vi "Day04-04_텍스트 파일 및 폴더 경로 설정.vi"() -> ()   [LabVIEW 2021]
uses:
  <vilib>/Utility/sysdir.llb/System Directory Type.ctl
panel:
  out "배열":dbl[][](array[numeric])
  out "텍스트 파일 열기 경로":path
  out "텍스트 파일 쓰기 경로":path
  out "파일 경로":path
  out "추가된 경로":path
  out "system directory":path caption="시스템 디렉토리"
  out "Application Directory":path caption="어플리케이션 디렉토리"
  out "경로":path
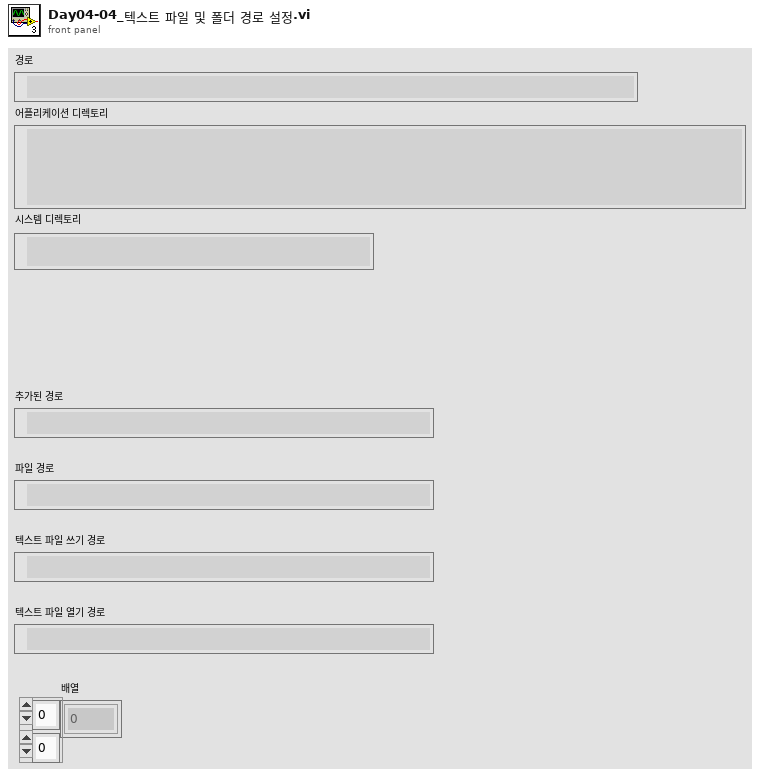
[diagram p1: front panel]
types:
  T1 = enum16{"open", "replace", "create", "open or create", "replace or create", "replace or create with confirmation"}
  T2 = typedef "System Directory Type.ctl" = i32
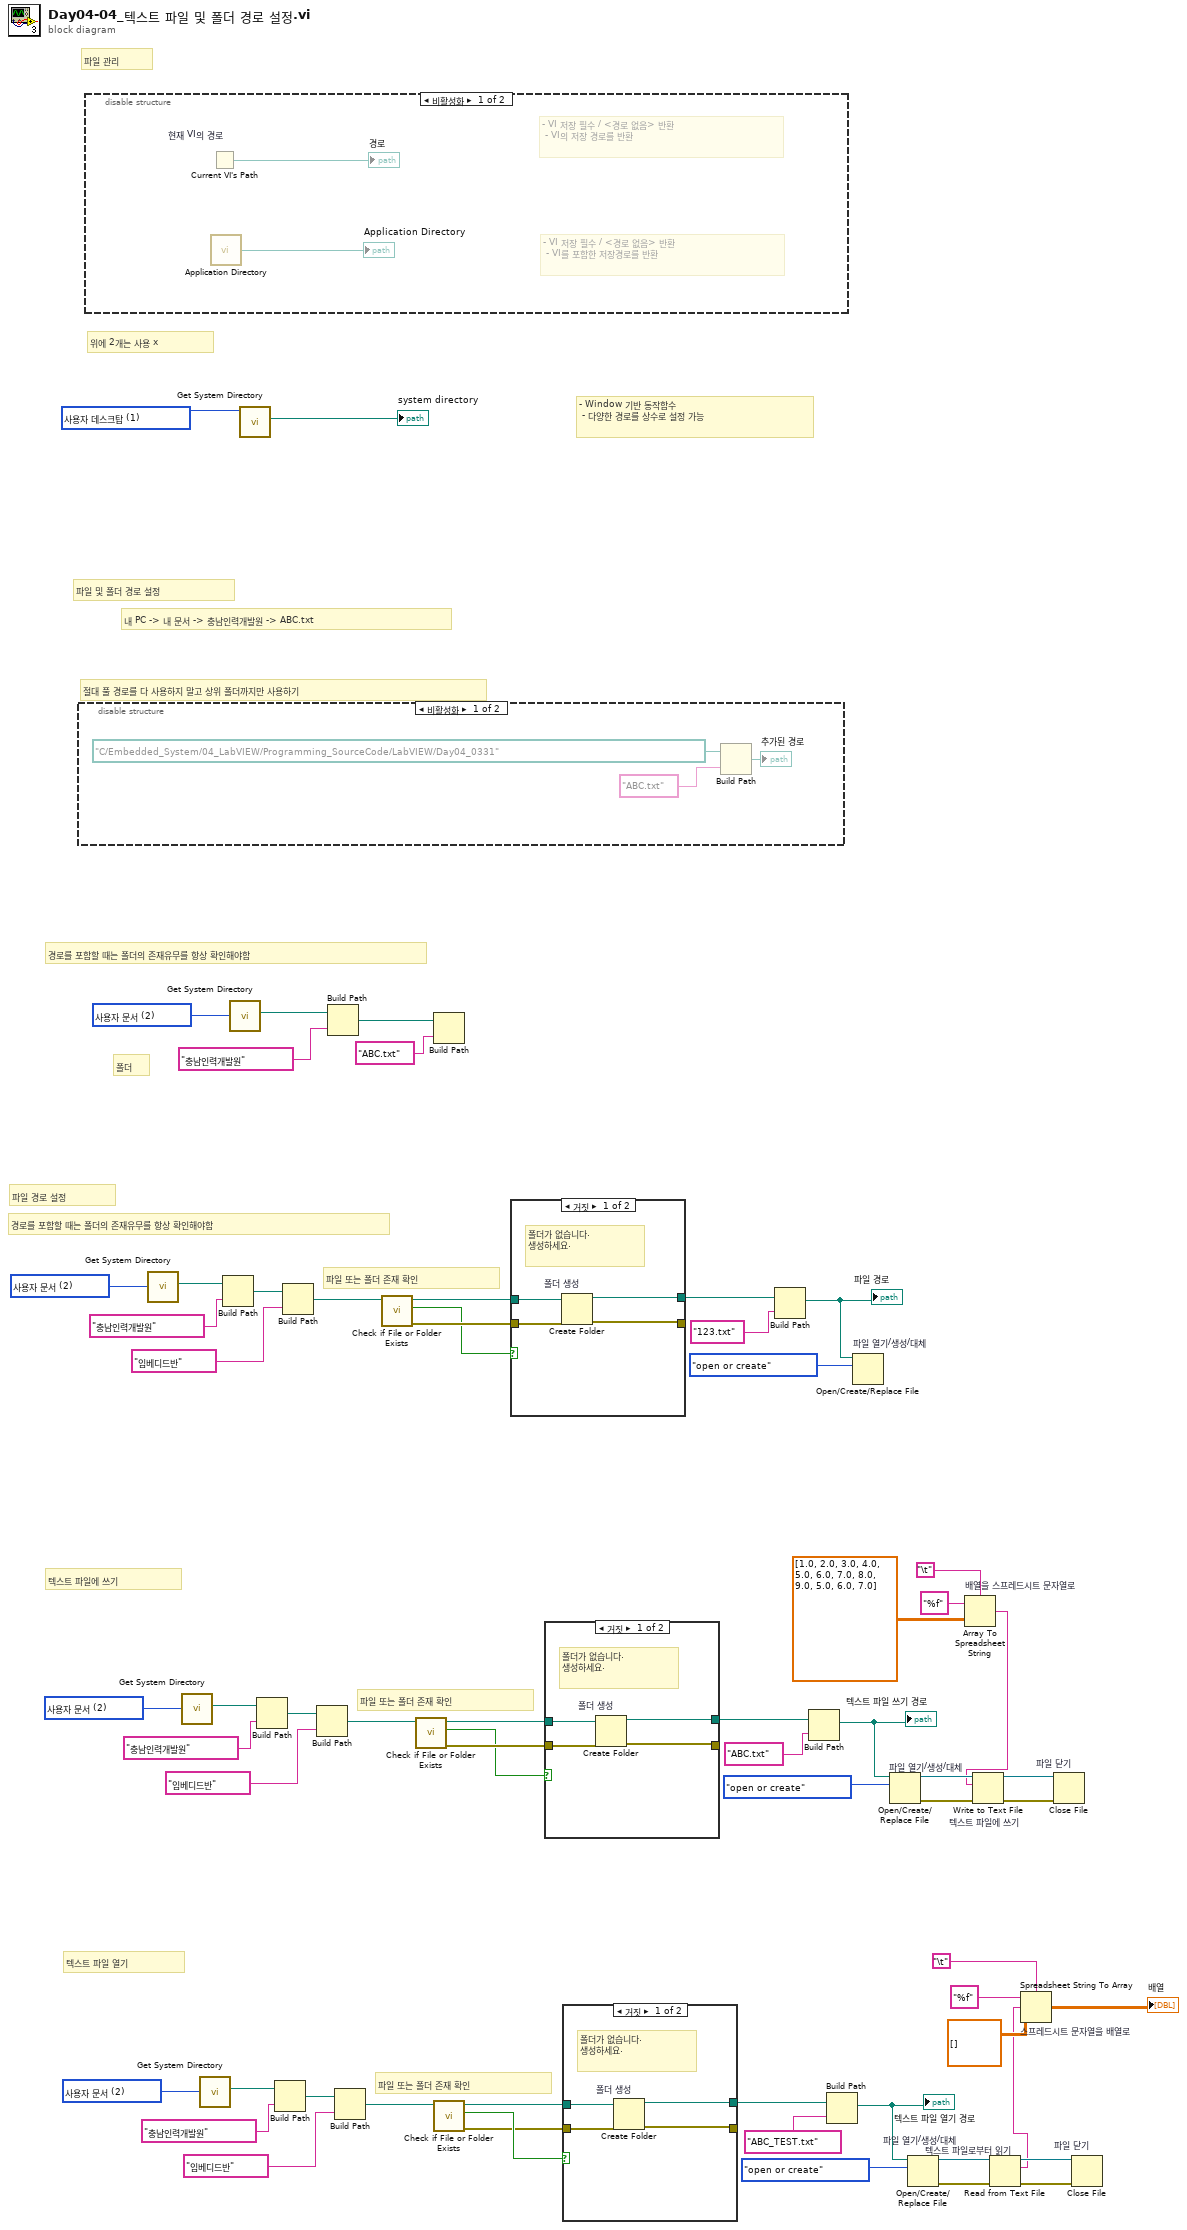
[diagram p0: block diagram]
diagram:
  w10 = T2 2 items=["사용자 홈"=0, "사용자 데스크탑"=1, "사용자 문서"=2, "사용자 어플리케이션 데이터"=3, "사용자 환경"=4, "사용자 임시"=5, "퍼블릭 문서"=6, "퍼블릭 어플리케이션 데이터"=7, "퍼블릭 환경"=8, "퍼블릭 캐시"=13, "시스템 코어 라이브러리"=9, "시스템 설치된 라이브러리"=10, "어플리케이션 파일"=11, "부팅 볼륨 루트"=12] ("system directory type")
  w43 = T2 2 items=["사용자 홈"=0, "사용자 데스크탑"=1, "사용자 문서"=2, "사용자 어플리케이션 데이터"=3, "사용자 환경"=4, "사용자 임시"=5, "퍼블릭 문서"=6, "퍼블릭 어플리케이션 데이터"=7, "퍼블릭 환경"=8, "퍼블릭 캐시"=13, "시스템 코어 라이브러리"=9, "시스템 설치된 라이브러리"=10, "어플리케이션 파일"=11, "부팅 볼륨 루트"=12] ("system directory type")
  w56 = T2 2 items=["사용자 홈"=0, "사용자 데스크탑"=1, "사용자 문서"=2, "사용자 어플리케이션 데이터"=3, "사용자 환경"=4, "사용자 임시"=5, "퍼블릭 문서"=6, "퍼블릭 어플리케이션 데이터"=7, "퍼블릭 환경"=8, "퍼블릭 캐시"=13, "시스템 코어 라이브러리"=9, "시스템 설치된 라이브러리"=10, "어플리케이션 파일"=11, "부팅 볼륨 루트"=12] ("system directory type")
  w61 = T2 2 items=["사용자 홈"=0, "사용자 데스크탑"=1, "사용자 문서"=2, "사용자 어플리케이션 데이터"=3, "사용자 환경"=4, "사용자 임시"=5, "퍼블릭 문서"=6, "퍼블릭 어플리케이션 데이터"=7, "퍼블릭 환경"=8, "퍼블릭 캐시"=13, "시스템 코어 라이브러리"=9, "시스템 설치된 라이브러리"=10, "어플리케이션 파일"=11, "부팅 볼륨 루트"=12] ("system directory type")
  w62 = T2 1 items=["사용자 홈"=0, "사용자 데스크탑"=1, "사용자 문서"=2, "사용자 어플리케이션 데이터"=3, "사용자 환경"=4, "사용자 임시"=5, "퍼블릭 문서"=6, "퍼블릭 어플리케이션 데이터"=7, "퍼블릭 환경"=8, "퍼블릭 캐시"=13, "시스템 코어 라이브러리"=9, "시스템 설치된 라이브러리"=10, "어플리케이션 파일"=11, "부팅 볼륨 루트"=12] ("system directory type")
  # "파일 또는 폴더 존재 확인"
  # "텍스트 파일 열기"
  # "파일 또는 폴더 존재 확인"
  # "텍스트 파일에 쓰기"
  # "파일 경로 설정"
  # "경로를 포함할 때는 폴더의 존재유무를 항상 확인해야함"
  # "파일 또는 폴더 존재 확인"
  # "폴더"
  # "경로를 포함할 때는 폴더의 존재유무를 항상 확인해야함"
  # "절대 풀 경로를 다 사용하지 말고 상위 폴더까지만 사용하기"
  # "내 PC -> 내 문서 -> 충남인력개발원 -> ABC.txt"
  # "파일 및 폴더 경로 설정"
  # "위에 2개는 사용 x"
  # "- Window 기반 동작함수\n - 다양한 경로를 상수로 설정 가능"
  # "파일 관리"
  n1 = disable-structure shown="비활성화" {
    frame Disabled {
      n2 = Build Path(base path=path "C:/Embedded_System/04_LabVIEW/Programming_SourceCode/LabVIEW/Day04_0331" ("이름 또는 상대 경로"), name or relative path="ABC.txt") -> (appended path=→"추가된 경로":path)
    }
    frame Enabled {
    }
  }
  n3 = disable-structure shown="비활성화" {
    frame Disabled {
      # "- VI 저장 필수 / <경로 없음> 반환\n - VI를 포함한 저장경로를 반환"
      # "- VI 저장 필수 / <경로 없음> 반환\n - VI의 저장 경로를 반환"
      n4 = Current VI's Path "현재 VI의 경로"() -> (path=→"경로":path)
      n5 = call <vilib>:"Application Directory.vi"() -> ("Application Directory"=→"Application Directory":path)
    }
    frame Enabled {
    }
  }
  n6 = call <vilib>:"Get System Directory.vi"("system directory type"=w56) -> ("system directory"=w55:path)  [unwired: 10 in]
  n7 = call <vilib>:"Get System Directory.vi"("system directory type"=w43) -> ("system directory"=w42:path)  [unwired: 10 in]
  n8 = call <vilib>:"Get System Directory.vi"("system directory type"=w10) -> ("system directory"=w11:path)  [unwired: 10 in]
  n9 = Build Path(base path=w55, name or relative path="충남인력개발원") -> (appended path=w46:path)
  n10 = call <vilib>:"Get System Directory.vi"("system directory type"=w61) -> ("system directory"=w60:path)  [unwired: 10 in]
  n11 = call <vilib>:"Get System Directory.vi"("system directory type"=w62) -> ("system directory"=→"system directory":path)  [unwired: 10 in]
  n12 = Build Path(base path=w42, name or relative path="충남인력개발원") -> (appended path=w33:path)
  n13 = Build Path(base path=w11, name or relative path="충남인력개발원") -> (appended path=w20:path)
  n14 = Build Path(base path=w46, name or relative path="임베디드반") -> (appended path=w44:path)
  n15 = Build Path(base path=w33, name or relative path="임베디드반") -> (appended path=w31:path)
  n16 = Build Path(base path=w60, name or relative path="충남인력개발원") -> (appended path=w58:path)
  n17 = Build Path(base path=w20, name or relative path="임베디드반") -> (appended path=w22:path)
  n18 = call <vilib>:"Check if File or Folder Exists.vi"("path"=w44) -> ("error out"=w52:errorcluster, "file or folder exists?"=w47:bool, "dup path"=w53:path)  [unwired: 8 in]
  n19 = call <vilib>:"Check if File or Folder Exists.vi"("path"=w31) -> ("error out"=w39:errorcluster, "file or folder exists?"=w34:bool, "dup path"=w40:path)  [unwired: 8 in]
  n20 = Build Path(base path=w58, name or relative path="ABC.txt") -> ()  [unwired: 1 out]
  n21 = call <vilib>:"Check if File or Folder Exists.vi"("path"=w22) -> ("error out"=w14:errorcluster, "file or folder exists?"=w19:bool, "dup path"=w13:path)  [unwired: 8 in]
  n22 = case shown="거짓" w47 {
    tunnel: w53 -> [w72 w74]
    tunnel: w52 -> [w71 w73]
    tunnel: [w70 w74] -> w50
    tunnel: [w69 w73] -> _
    frame False {
      # "폴더가 없습니다.\n생성하세요."
      n23 = Create Folder "폴더 생성"(path (use dialog)=w72, error in=w71) -> (created path=w70:path, error out=w69:errorcluster)  [unwired: 1 in, 1 out]
    }
    frame True {
    }
  }
  n24 = case shown="거짓" w34 {
    tunnel: w40 -> [w78 w80]
    tunnel: w39 -> [w77 w79]
    tunnel: [w76 w80] -> w37
    tunnel: [w75 w79] -> _
    frame False {
      # "폴더가 없습니다.\n생성하세요."
      n25 = Create Folder "폴더 생성"(path (use dialog)=w78, error in=w77) -> (created path=w76:path, error out=w75:errorcluster)  [unwired: 1 in, 1 out]
    }
    frame True {
    }
  }
  n26 = case shown="거짓" w19 {
    tunnel: w13 -> [w84 w86]
    tunnel: w14 -> [w83 w85]
    tunnel: [w82 w86] -> w16
    tunnel: [w81 w85] -> _
    frame False {
      # "폴더가 없습니다.\n생성하세요."
      n27 = Create Folder "폴더 생성"(path (use dialog)=w84, error in=w83) -> (created path=w82:path, error out=w81:errorcluster)  [unwired: 1 in, 1 out]
    }
    frame True {
    }
  }
  n28 = Build Path(base path=w50, name or relative path="123.txt") -> (appended path=w49:path)
  "파일 경로" <- w49
  n29 = Build Path(base path=w37, name or relative path="ABC.txt") -> (appended path=w36:path)
  "텍스트 파일 쓰기 경로" <- w36
  n30 = Build Path(base path=w16, name or relative path="ABC_TEST.txt") -> (appended path=w17:path)
  "텍스트 파일 열기 경로" <- w17
  n31 = Open/Create/Replace File "파일 열기/생성/대체"(file path (use dialog)=w49, operation (0:open)=T1."open or create" ("동작(0:open)")) -> ()  [unwired: 4 in, 3 out]
  n32 = Open/Create/Replace File "파일 열기/생성/대체"(file path (use dialog)=w36, operation (0:open)=T1."open or create" ("동작(0:open)")) -> (refnum out=w30:refnum<file>, error out=w28:errorcluster)  [unwired: 4 in, 1 out]
  n33 = Open/Create/Replace File "파일 열기/생성/대체"(file path (use dialog)=w17, operation (0:open)=T1."open or create" ("동작(0:open)")) -> (refnum out=w6:refnum<file>, error out=w5:errorcluster)  [unwired: 4 in, 1 out]
  n34 = Array To Spreadsheet String "배열을 스프레드시트 문자열로"(delimiter (Tab)="\t", array=dbl[][] [[1.0, 2.0, 3.0], [4.0, 5.0, 6.0], [7.0, 8.0, 9.0], [5.0, 6.0, 7.0]], 3:"%f" ("포맷 문자열")) -> (spreadsheet string=w23:string)
  n35 = Write to Text File "텍스트 파일에 쓰기"(file (use dialog)=w30, text=w23, error in=w28) -> (refnum out=w29:refnum<file>, error out=w27:errorcluster)  [unwired: 1 in, 1 out]
  n36 = Read from Text File "텍스트 파일로부터 읽기"(file (use dialog)=w6, error in=w5) -> (refnum out=w4:refnum<file>, text=w2:string, error out=w3:errorcluster)  [unwired: 2 in, 1 out]
  n37 = Spreadsheet String To Array "스프레드시트 문자열을 배열로"(delimiter (Tab)="\t", format string="%f" ("포맷 문자열"), spreadsheet string=w2, array type (2D Dbl)=dbl[][] [] ("배열 타입(2D Dbl)")) -> (array=→"배열":dbl[][])
  n38 = Close File "파일 닫기"(refnum=w29, error in=w27) -> ()  [unwired: 2 out]
  n39 = Close File "파일 닫기"(refnum=w4, error in=w3) -> ()  [unwired: 2 out]
